vi "Init.vi"(8 "error in (no error)":errorcluster, 10 "HAL GOOP4.lvlib:Study Base.lvclass":refnum<class "Series Base.lvclass">, 11 "Series Actor in":refnum<class "Series Actor.lvclass">) -> (0 "error out":errorcluster, 3 "Series Actor out":refnum<class "Series Actor.lvclass">)   [LabVIEW 2023, in "Series Actor.lvlib" / "Series Actor.lvclass"]
uses:
  Series Actor.lvclass
  C:/Program Files/National Instruments/LabVIEW 2023/vi.lib/ActorFramework/Actor/Actor.lvclass
  Series Base/Series Base.lvclass
  Series Base/Series Base.lvclass/Series Base.ctl
  <vilib>/ActorFramework/Message Enqueuer/Message Enqueuer.lvclass
  Task/Task Actor/Task Actor/Task Actor/Task Actor.lvclass
  Series Actor.lvclass/Series Actor.ctl
  Task/Task Actor/Task Actor/Task Actor/Task Actor.lvclass/Task Actor.ctl
  <vilib>/ActorFramework/Actor/Actor.lvclass
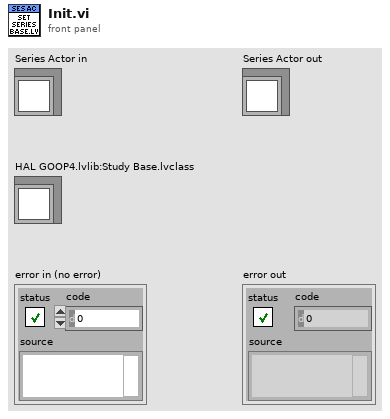
[diagram p1: front panel]
types:
  T1 = map{string, refnum<class "Message Enqueuer.lvclass">}
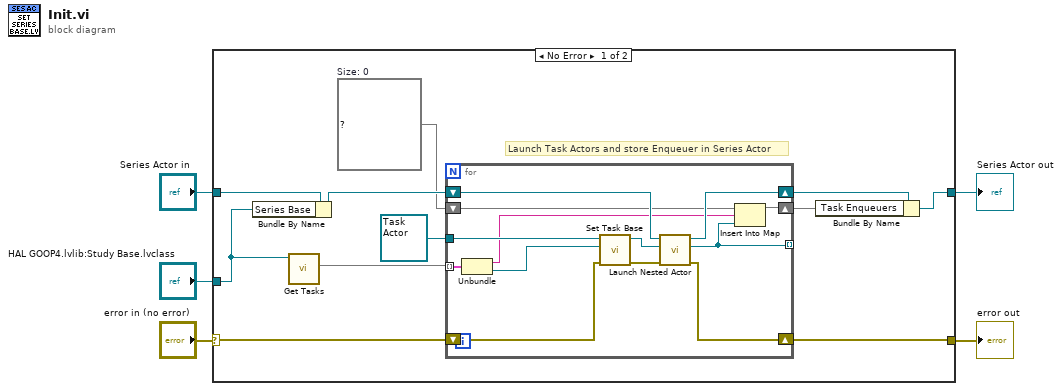
[diagram p0: block diagram]
diagram:
  n1 = case shown="No Error" "error in (no error)" {
    selector: "error in (no error)" -> [w9 w31]
    tunnel: "Series Actor in" -> [w16 w30]
    tunnel: [w8 w30] -> w4
    tunnel: "HAL GOOP4.lvlib:Study Base.lvclass" -> [w10 _]
    tunnel: [w6 w31] -> w1
    frame No Error {
      w7 = T1 {}  # Size: 0
      # "Launch Task Actors and store Enqueuer in Series Actor"
      n2 = Bundle By Name(cluster=w16, "Series Base"=w10) -> (w11:refnum<class "Series Actor.lvclass">)
      n3 = call "Get Tasks.vi"("HAL GOOP4:Series Base in"=w10) -> ("Tasks"=w15:map{string, refnum<class "Task Base.lvclass">})  [unwired: 8 in, 2 out]
      n4 = for {
        tunnel: w15 -> [w19] mode=indexing
        shift-right: [w23] -> w13
        shift-left: w11 -> [w29]
        tunnel: refnum<class "Task Actor.lvclass"> refnum ("Task Actor.lvlib:Task Actor.lvclass") -> [w28]
        shift-right: [w24] -> w6
        shift-left: w9 -> [w26]
        shift-right: [w21] -> w12
        shift-left: w7 -> [w22]
        tunnel: [w20] -> _ mode=indexing
        n5 = Unbundle(w19) -> (w18:string, "Task"=w17:refnum<class "Task Base.lvclass">)
        n6 = call "Set Task Base.vi"("error in (no error)"=w26, "HAL GOOP4.lvlib:Task Base.lvclass"=w17, "Task Actor in"=w28) -> ("error out"=w25:errorcluster, "Task Actor out"=w27:refnum<class "Task Actor.lvclass">)  [unwired: 7 in]
        n7 = call <vilib>:"Launch Nested Actor.vi"("error in (no error)"=w25, "Nested Actor"=w27, "Caller Actor in"=w29) -> ("error out"=w24:errorcluster, "Nested Actor's Enqueuer"=w20:refnum<class "Message Enqueuer.lvclass">, "Caller Actor out"=w23:refnum<class "Series Actor.lvclass">)  [unwired: 6 in]
        n8 = Insert Into Map(map in=w22, key=w18, value=w20) -> (map out=w21:T1)  [unwired: 2 out]
      }
      n9 = Bundle By Name(cluster=w13, "Task Enqueuers"=w12) -> (w8:refnum<class "Series Actor.lvclass">)
    }
    frame Error {
    }
  }
  "error out" <- w1
  "Series Actor out" <- w4
